vi "merFISH_save_path_definition.vi"(0 "merFISH path":path, 1 "List probe Refnum":refnum<vi>, 2 "Data":T1, 3 "error in":errorcluster) -> (4 "Acquisition_parameters path":path, 5 "Z_position_file path":path, 6 "Movie path":path, 7 "error out":errorcluster)   [LabVIEW 2015]
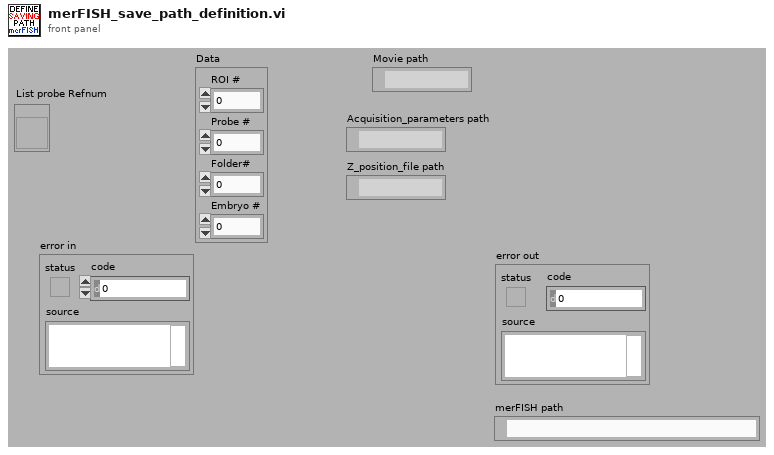
[diagram p1: front panel]
types:
  T1 = cluster{"ROI #":i32, "Probe #":i32, "Folder# ":i32, "Embryo #":i32}
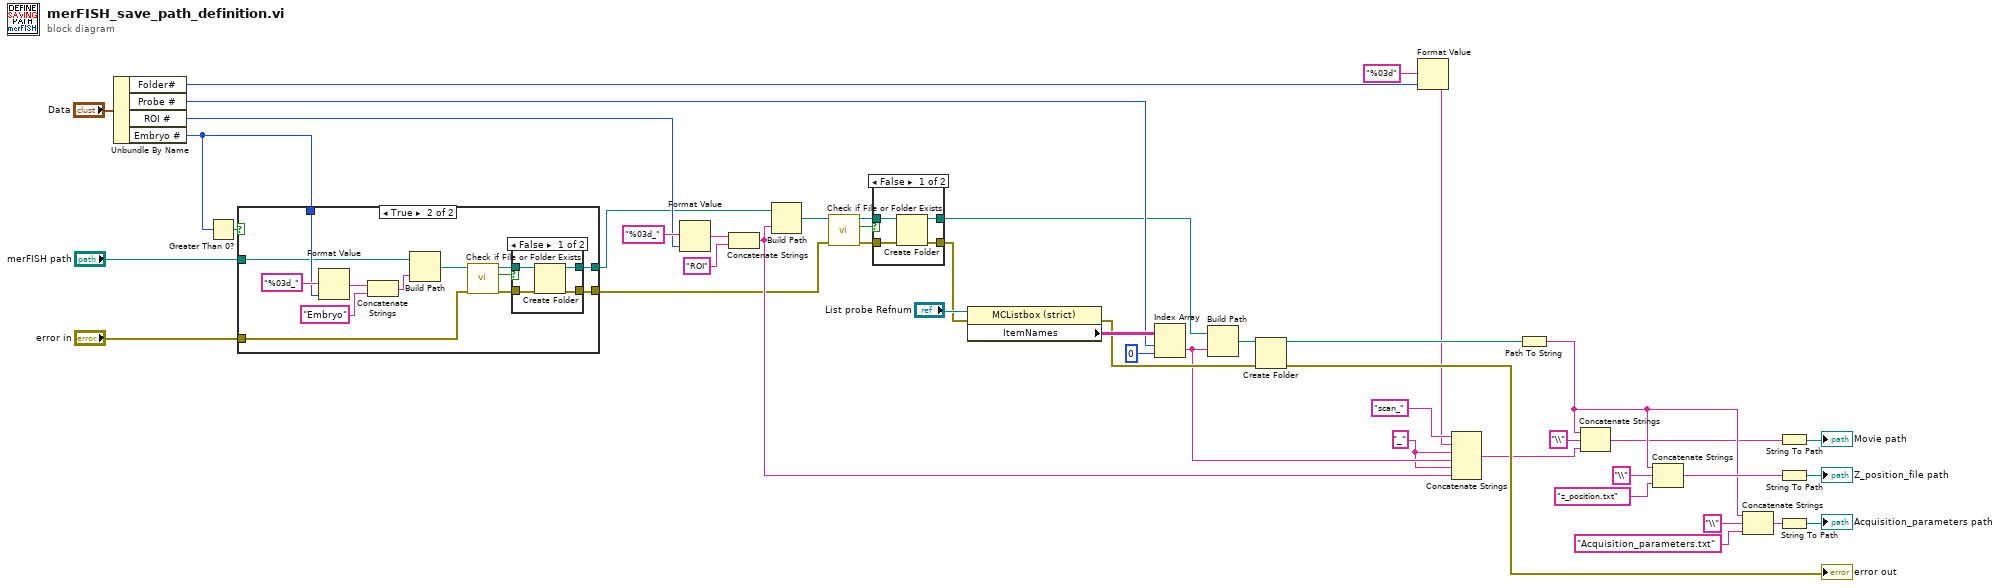
[diagram p0: block diagram]
diagram:
  w15 = "_" ("string")
  n1 = Unbundle By Name("Data") -> ("Folder#"=w13:i32, "Probe #"=w27:i32, "ROI #"=w34:i32, "Embryo #"=w3:i32)
  n2 = Greater Than 0?(x=w3) -> (x > 0?=w4:bool)
  n3 = case shown="True" w4 {
    tunnel: w3 -> [_ w52]
    tunnel: "error in" -> [w46 w51]
    tunnel: [w46 w50] -> w5
    tunnel: "merFISH path" -> [w47 w49]
    tunnel: [w47 w48] -> w1
    frame False {
    }
    frame True {
      n4 = Format Value(format string="%03d_" ("string (\"\")"), value (0)=w52) -> (output string=w54:string)  [unwired: 1 in]
      n5 = Concatenate Strings(w54, "Embryo" ("string")) -> (w60:string)
      n6 = Build Path(base path=w49, name or relative path=w60) -> (appended path=w56:path)
      n7 = call <vilib>:"Check if File or Folder Exists.vi"("error in (no error)"=w51, "path"=w56) -> ("error out"=w58:errorcluster, "file or folder exists?"=w57:bool, "dup path"=w59:path)  [unwired: 7 in]
      n8 = case shown="False" w57 {
        tunnel: w58 -> [w64 w65]
        tunnel: w59 -> [w63 w66]
        tunnel: [w62 w65] -> w50
        tunnel: [w61 w66] -> w48
        frame False {
          n9 = Create Folder(path (use dialog)=w63, error in=w64) -> (created path=w61:path, error out=w62:errorcluster)  [unwired: 1 in, 1 out]
        }
        frame True {
        }
      }
    }
  }
  n10 = Format Value(format string="%03d_" ("string (\"\")"), value (0)=w34) -> (output string=w39:string)  [unwired: 1 in]
  n11 = Concatenate Strings(w39, "ROI" ("string")) -> (w18:string)
  n12 = Build Path(base path=w1, name or relative path=w18) -> (appended path=w25:path)
  n13 = call <vilib>:"Check if File or Folder Exists.vi"("error in (no error)"=w5, "path"=w25) -> ("error out"=w23:errorcluster, "file or folder exists?"=w24:bool, "dup path"=w22:path)  [unwired: 7 in]
  n14 = case shown="False" w24 {
    tunnel: w23 -> [w70 w71]
    tunnel: w22 -> [w69 w72]
    tunnel: [w68 w71] -> w21
    tunnel: [w67 w72] -> w20
    frame False {
      n15 = Create Folder(path (use dialog)=w69, error in=w70) -> (created path=w67:path, error out=w68:errorcluster)  [unwired: 1 in, 1 out]
    }
    frame True {
    }
  }
  n16 = property class="MCListbox (strict)"(reference="List probe Refnum", error in=w21) -> (error out=w30:errorcluster, "ItemNames"=w32:string[][])  [unwired: 1 out]
  n17 = Index Array(array=w32, index (row)=w27, index (col)=0 ("index (row)")) -> (element=w19:string)
  n18 = Build Path(base path=w20, name or relative path=w19) -> (appended path=w31:path)
  n19 = Create Folder(path (use dialog)=w31, error in=w30) -> (created path=w28:path, error out=→"error out":errorcluster)  [unwired: 1 in, 1 out]
  n20 = Format Value(format string="%03d" ("string (\"\")"), value (0)=w13) -> (output string=w12:string)  [unwired: 1 in]
  n21 = Concatenate Strings("scan_" ("string"), w12, w15, w19, w15, w18) -> (w17:string)
  n22 = Path To String(path=w28) -> (string=w36:string)
  n23 = Concatenate Strings(w36, "\\" ("string"), w17) -> (w11:string)
  n24 = Concatenate Strings(w36, "\\" ("string"), "z_position.txt" ("string")) -> (w43:string)
  n25 = Concatenate Strings(w36, "\\" ("string"), "Acquisition_parameters.txt" ("string")) -> (w42:string)
  n26 = String To Path(string=w11) -> (path=→"Movie path":path)
  n27 = String To Path(string=w43) -> (path=→"Z_position_file path":path)
  n28 = String To Path(string=w42) -> (path=→"Acquisition_parameters path":path)
